vi "L Vwrite read async serial.vi"(7 "bsize":i32, 9 "buf":i8[](array[numeric])=array[4097 elements], 10 "iswrite":i32, 11 "h":u32) -> (1 "buf out":i8[](array[numeric]), 3 "function return":i32)   [LabVIEW 2010]
doc: "int LVwrite_read_async_serial(pserial_handle_t h, int iswrite,void*buf,int bsize);"
uses:
  <userlib>/libcommon_serial/libcommon_serial.so
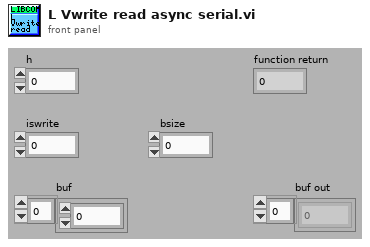
[diagram p1: front panel]
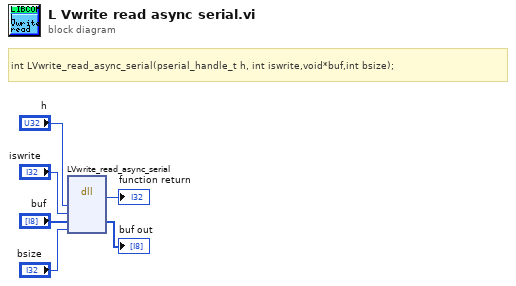
[diagram p0: block diagram]
diagram:
  # "int LVwrite_read_async_serial(pserial_handle_t h, int iswrite,void*buf,int bsize);"
  n1 = dll-call lib="usr/local/natinst/LabVIEW-2010/user.lib/libcommon_serial/libcommon_serial.*" fn="LVwrite_read_async_serial"("h"="h", "iswrite"="iswrite", "buf"="buf", "bsize"="bsize") -> (→"function return":i32, "buf"=→"buf out":i8[])  [unwired: 6 in, 2 out]
